vi "Check For Internet Connection to WIKI.vi"() -> (0 "error out":errorcluster, 2 "Connected to internet?":bool)   [LabVIEW 2015]
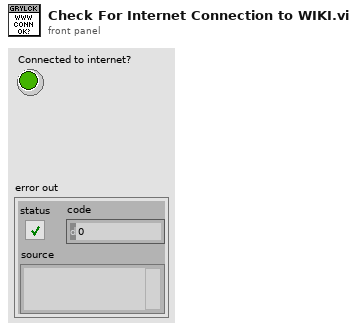
[diagram p1: front panel]
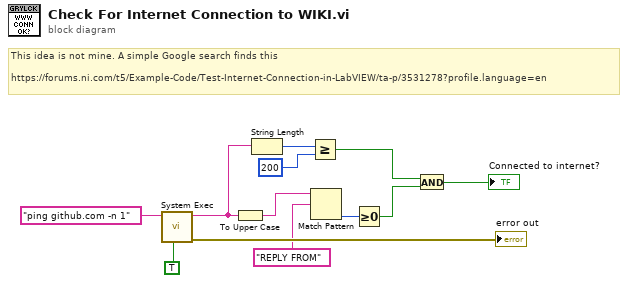
[diagram p0: block diagram]
diagram:
  # "This idea is not mine. A simple Google search finds this\n\nhttps://forums.ni.com/t5/Example-Code/Test-Internet-Connection-in-LabVIEW/ta-p/3531278?profile.language=en"
  n1 = call <vilib>:"System Exec.vi"("run minimized? (F)"=TRUE, "command line"="ping github.com -n 1") -> ("error out"=→"error out":errorcluster, "standard output"=w7:string)  [unwired: 6 in, 2 out]
  n2 = To Upper Case(1:w7) -> (0:w6:string)
  n3 = String Length(string=w7) -> (length=w12:i32)
  n4 = Greater Or Equal?(x=w12, y=200) -> (x >= y?=w3:bool)
  n5 = Match Pattern(string=w6, regular expression="REPLY FROM") -> (offset past match=w4:i32)  [unwired: 1 in, 3 out]
  n6 = Greater Or Equal To 0?(x=w4) -> (x >= 0?=w2:bool)
  n7 = And(x=w3, y=w2) -> (x .and. y?=→"Connected to internet?":bool)
